vi "DllFxpExpTemp.vi"(6 "ready for output":bool, 9 "input valid":bool, 11 "phase":fxp<+,1,1>) -> (1 "output valid":bool, 3 "Exp":fxp<+,1,1>, 4 "ready for input":bool)   [LabVIEW 2017]
uses:
  <vilib>/rvi/FXPMathLib/FxpExp/subVIs/nifxpmath_Exp_SimConfig.ctl
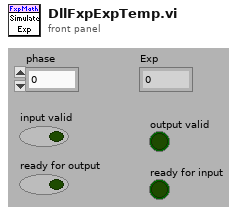
[diagram p1: front panel]
types:
  T1 = typedef "nifxpmath_Exp_SimConfig.ctl" = cluster{"kPhaseLen":u16, "kPhaseIwl":i16, "kPhaseSigned":bool, "kInputRegister":bool, "kOutputRegister":bool, "kExpLen":u16, "kPrecision":u16, "kIteration":u16, "QuantiMode":u16, "HandShake":bool, "CycleLimit":u16, "StrictLimit":bool}
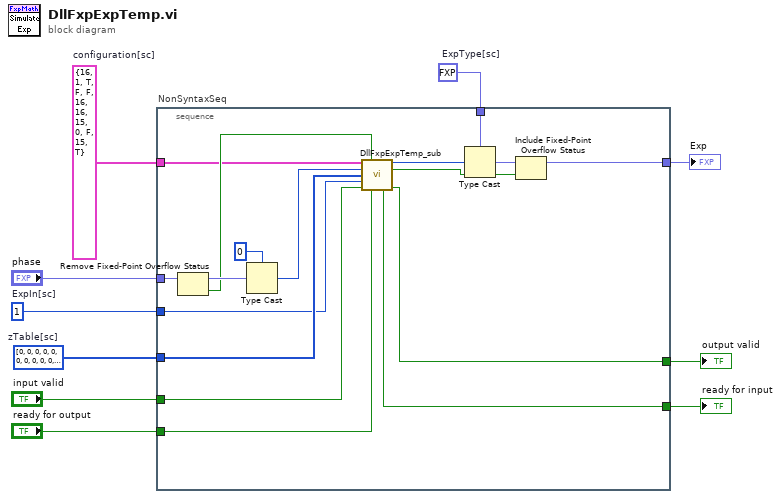
[diagram p0: block diagram]
diagram:
  w1 = T1 {"kPhaseLen"=16, "kPhaseIwl"=1, "kPhaseSigned"=TRUE, "kInputRegister"=FALSE, "kOutputRegister"=FALSE, "kExpLen"=16, "kPrecision"=16, "kIteration"=15, "QuantiMode"=0, "HandShake"=FALSE, "CycleLimit"=15, "StrictLimit"=TRUE}  # configuration[sc]
  w4 = u64 1  # ExpIn[sc]
  w5 = fxp<+,1,1> 0.0  # ExpType[sc]
  w7 = u64[] [0, 0, 0, 0, 0, 0, 0, 0, 0, 0, 0, 0, 0, 0, 0, 0]  # zTable[sc]
  n1 = stacked-sequence "NonSyntaxSeq" {
    tunnel: "phase" -> [w27]
    tunnel: "input valid" -> [w17]
    tunnel: [w22] -> w2
    tunnel: [w14] -> w9
    tunnel: [w13] -> w8
    tunnel: w1 -> [w11]
    tunnel: w4 -> [w18]
    tunnel: w7 -> [w19]
    tunnel: w5 -> [w25]
    tunnel: "ready for output" -> [w16]
    frame #0 {
      n2 = Remove Fixed-Point Overflow Status(3:w27) -> (0:w20:bool, 1:w23:fxp<+,1,1>)
      n3 = Type Cast(type=u64 0, x=w23) -> (*(type *) &x=w21:u64)
      n4 = call <vilib>:"DllFxpExpTemp_sub.vi"("configuration[sc]"=w11, "phase ovfl status"=w20, "phase"=w21, "zTable"=w19, "exp initial"=w18, "input valid"=w17, "ready for output"=w16) -> ("exp"=w15:u64, "exp ovfl status"=w12:bool, "ready for input"=w13:bool, "output valid"=w14:bool)  [unwired: 5 out]
      n5 = Type Cast(type=w25, x=w15) -> (*(type *) &x=w24:fxp<+,1,1>)
      n6 = Include Fixed-Point Overflow Status(2:w12, 3:w24) -> (1:w22:fxp<+,1,1>)
    }
  }
  "Exp" <- w2
  "output valid" <- w9
  "ready for input" <- w8
